vi "read_data.vi"(8 "error in (no error)":errorcluster, 11 "DAQ_DL091205Readers in":refnum<class "DAQ_DL091205Readers.lvclass">) -> (0 "error out":errorcluster, 2 "finished?":bool, 3 "DAQ_DL091205Readers out":refnum<class "DAQ_DL091205Readers.lvclass">, 4 "buffer overflow?":bool)   [LabVIEW 2010, in "DAQ_DL091205Readers.lvclass"]
doc: "This VI reads data sampless from [1..n] SignalReaders. Each SignalReader represents a distinct physical device."
uses:
  DAQ_DL091205Readers.lvclass
  DAQ_DL091205Readers.lvclass/DAQ_DL091205Readers.ctl
  SignalReader/GenericSignalReader/GenericSignalReader/GenericSignalReader.lvclass
  DAQ_DL090211Scaffold/DAQ_DL090211Scaffold/DAQ_DL090211Scaffold.lvclass
  ImagingMode/GenericImagingMode/GenericImagingMode/trigger_enum.ctl
  ImagingMode/GenericImagingMode/GenericImagingMode/GenericImagingMode.lvclass
  common/classes/ErrorController/ErrorController/class_data.vi
  common/classes/ErrorController/ErrorController/ErrorController.lvclass
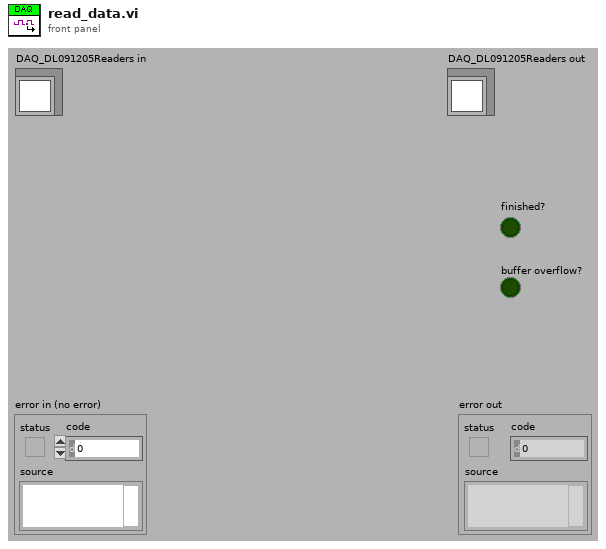
[diagram p1: front panel]
types:
  T1 = typedef "GenericImagingMode.lvclass/trigger_enum.ctl" = enum16{"NULL", "proceed"}
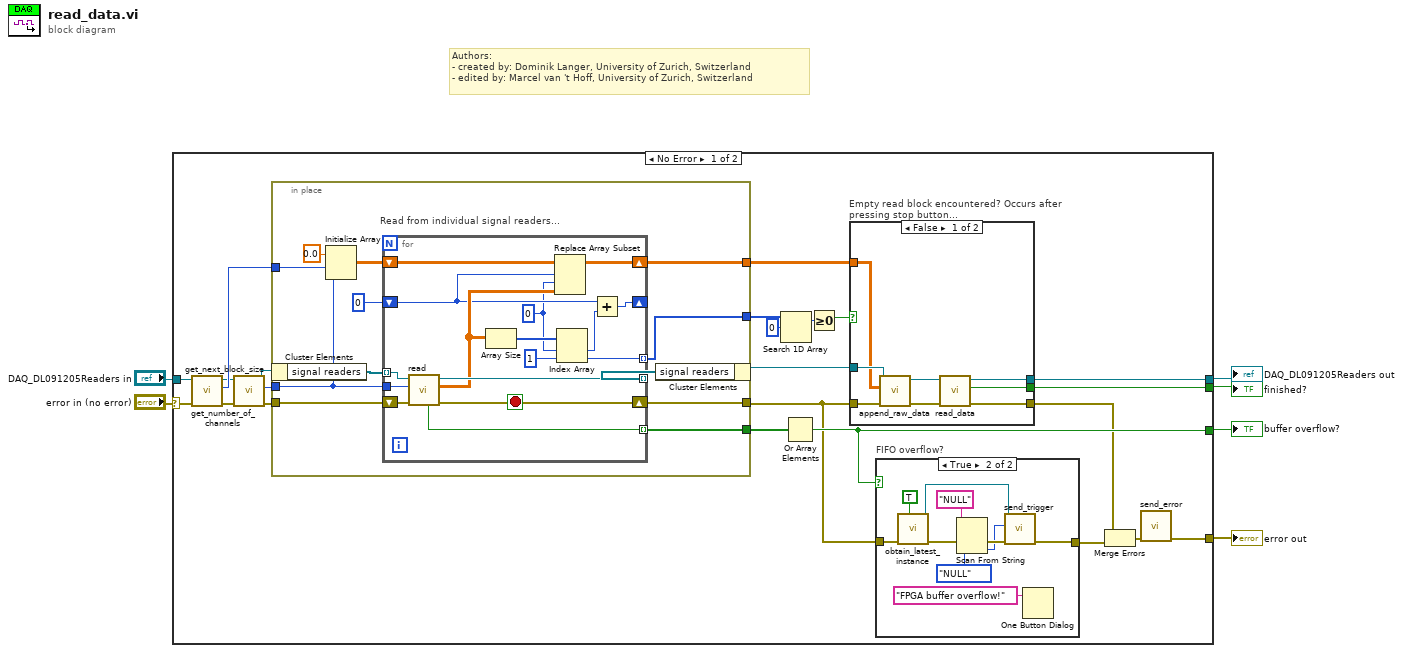
[diagram p0: block diagram]
diagram:
  # "Authors: \n- created by: Dominik Langer, University of Zurich, Switzerland\n- edited by: Marcel van 't Hoff, University of Zurich, Switzerland"
  n1 = case shown="No Error" "error in (no error)" {
    selector: "error in (no error)" -> [w15 w80]
    tunnel: [w23 w80] -> w6
    tunnel: "DAQ_DL091205Readers in" -> [w14 w79]
    tunnel: [w29 w79] -> w4
    tunnel: [w28 _] -> w3
    tunnel: [w27 _] -> w5
    frame No Error {
      n2 = call-dynamic "get_number_of_channels.vi"("error in (no error)"=w15, "GenericDAQ.lvclass in"=w14) -> ("error out"=w13:errorcluster, "number of channels"=w18:i32, "GenericDAQ.lvclass out"=w16:refnum<class "DAQ_DL091205Readers.lvclass">)  [unwired: 7 in]
      n3 = call-dynamic "get_next_block_size.vi"("error in (no error)"=w13, "GenericDAQ in"=w16) -> ("error out"=w22:errorcluster, "current block size"=w17:i32, "GenericDAQ out"=w19:refnum<class "DAQ_DL091205Readers.lvclass">)  [unwired: 7 out]
      n4 = in-place {
        in-place-border: w17 -> [w43]
        in-place-border: w22 -> [w50]
        in-place-border: [w49] -> w11
        in-place-border: [w47] -> w21
        in-place-border: [w46] -> w12
        in-place-border: w18 -> [w41]
        in-place-border: [w40] -> w9
        n5 = in-place-cluster #1(w19) -> ("signal readers"=w51:refnum<class "GenericSignalReader.lvclass">[])
        n6 = Initialize Array(0.0, w41, w43) -> (w44:dbl[][])
        n7 = for "Read from individual signal readers..." {
          tunnel: w51 -> [w66] mode=indexing
          tunnel: [w65] -> w48 mode=indexing
          tunnel: w43 -> [w64]
          shift-right: [w61] -> w46
          shift-left: w44 -> [w62]
          tunnel: [w63] -> w47 mode=indexing
          shift-right: [w60] -> w49
          shift-left: w50 -> [w67]
          shift-right: [w58] -> _
          shift-left: 0 -> [w55]
          tunnel: [w52] -> w40 mode=indexing
          stop <- w60 stop-if-true
          w54 = 0 ("index")
          n8 = call-dynamic "read.vi"("error in (no error)"=w67, "block size"=w64, "SignalReader in"=w66) -> ("error out"=w60:errorcluster, "signals read"=w59:dbl[][], "SignalReader out"=w65:refnum<class "GenericSignalReader.lvclass">, "buffer overflow?"=w63:bool)  [unwired: 4 in, 1 out]
          n9 = Array Size(array=w59) -> (size(s)=w57:i32[])
          n10 = Replace Array Subset(array=w62, new element=w59, index (row)=w55, index (col)=w54) -> (w61:dbl[][])
          n11 = Index Array(array=w57, index #1=w54, index #2=1 ("index")) -> (element #1=w56:i32, element #2=w52:i32)
          n12 = Add(x=w55, y=w56) -> (x+y=w58:i32)
        }
        n13 = in-place-cluster #1("signal readers"=w48) -> (w20:refnum<class "DAQ_DL091205Readers.lvclass">)
      }
      n14 = Search 1D Array(1D array=w9, element=0) -> (index of element=w8:i32)  [unwired: 1 in]
      n15 = Or Array Elements(Boolean array=w21) -> (logical OR=w27:bool)
      n16 = Greater Or Equal To 0?(x=w8) -> (x >= 0?=w7:bool)
      n17 = case "Empty read block encountered? Occurs after pressing stop button..." shown="False" w7 {
        tunnel: [w37 w39] -> w29
        tunnel: [w36 _] -> w28
        tunnel: [w35 w38] -> w25
        tunnel: w20 -> [w34 w39]
        tunnel: w12 -> [w31 _]
        tunnel: w11 -> [w30 w38]
        frame False {
          n18 = call-dynamic "append_raw_data.vi"("error in (no error)"=w30, "channels raw data block"=w31, "GenericDAQ in"=w34) -> ("error out"=w33:errorcluster, "GenericDAQ out"=w32:refnum<class "DAQ_DL091205Readers.lvclass">)  [unwired: 7 out]
          n19 = call-parent "read_data.vi"("error in (no error)"=w33, "GenericDAQ in"=w32) -> ("error out"=w35:errorcluster, "finished?"=w36:bool, "GenericDAQ out"=w37:refnum<class "DAQ_DL091205Readers.lvclass">)  [unwired: 6 in, 1 out]
        }
        frame True {
        }
      }
      n20 = case "FIFO overflow?" shown="True" w27 {
        tunnel: w11 -> [w68 w77]
        tunnel: [w68 w76] -> w26
        frame False {
        }
        frame True {
          n21 = call "obtain_latest_instance.vi"("quick, but maybe outdated?"=TRUE, "error in (no error)"=w77) -> ("error out"=w73:errorcluster, "GenericScanMode out"=w75:refnum<class "GenericImagingMode.lvclass">)  [unwired: 8 in]
          n22 = Scan From String(input string="NULL", error in=w73, default 1=trigger_enum."NULL" ("message")) -> (error out=w72:errorcluster, output 1=w69:T1)  [unwired: 2 in, 2 out]
          n23 = call-dynamic "send_trigger.vi"("error in (no error)"=w72, "message"=w69, "GenericScanMode in"=w75) -> ("error out"=w76:errorcluster)  [unwired: 7 in, 1 out]
          n24 = One Button Dialog(message="FPGA buffer overflow!") -> ()  [unwired: 2 out]
        }
      }
      n25 = Merge Errors(w25, w26) -> (w24:errorcluster)
      n26 = call "send_error.vi"("error in (no error)"=w24) -> ("error out"=w23:errorcluster)  [unwired: 10 in]
    }
    frame Error {
    }
  }
  "error out" <- w6
  "DAQ_DL091205Readers out" <- w4
  "finished?" <- w3
  "buffer overflow?" <- w5
